vi "前面板对象常用属性.vi"() -> ()   [LabVIEW 2010]
panel:
  out "1号罐图标大小":cluster{"宽":u32, "高":u32}
  in  "停止":bool
  in  "键盘焦点":bool
  in  "极限设定":dbl(slide)=5.252525252525253 scale=0.0..10.0
  out "4号罐液位":dbl(slide)=6.506024096385542 scale=0.0..10.0
  in  "可用":i32(listbox)
  in  "3号罐液位":dbl(slide)=6.506024096385542 scale=0.0..10.0
  in  "不闪烁   闪烁":bool=TRUE
  in  "2号罐液位":dbl(slide)=6.385542168674699 scale=0.0..10.0
  in  "1号罐液位":dbl(slide)=6.265060240963855 scale=0.0..10.0
  in  "不可见   可见":bool=TRUE
  # "取消    设定"
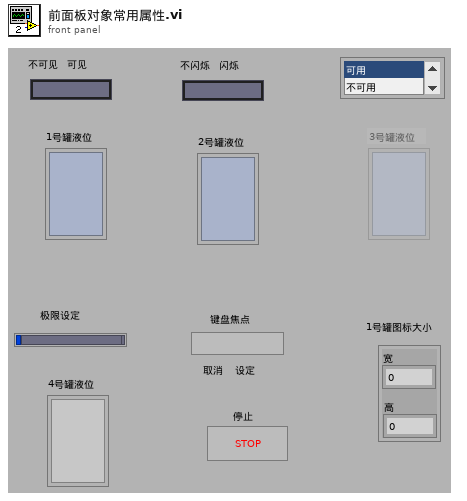
[diagram p1: front panel]
types:
  T1 = typedef "LVBoundsTypeDef.ctl" = cluster{"Width":u32, "Height":u32}
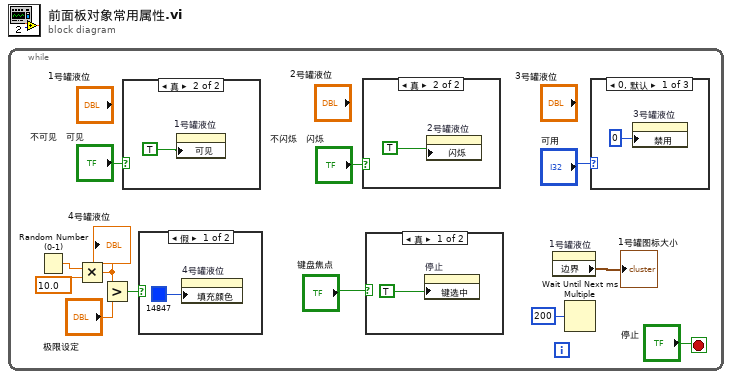
[diagram p0: block diagram]
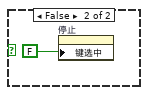
[diagram p2: hidden frame]
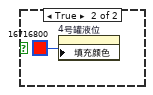
[diagram p3: hidden frame]
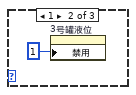
[diagram p4: hidden frame]
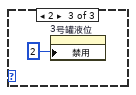
[diagram p5: hidden frame]
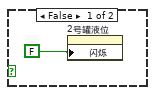
[diagram p6: hidden frame]
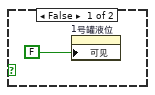
[diagram p7: hidden frame]
diagram:
  n1 = while {
    stop <- "停止" stop-if-true
    n2 = Random Number (0-1)() -> (number: 0 to 1=w7:dbl)
    n3 = Multiply(x=w7, y=10.0) -> (x*y=w5:dbl)
    "4号罐液位" <- w5
    n4 = Greater?(x=w5, y="极限设定") -> (0:w8:bool)
    n5 = case shown="真" "不可见   可见" {
      frame False {
        n6 = property on="1号罐液位" class="Slide (严格)"("可见"=FALSE) -> ()  [unwired: 2 in, 2 out]
      }
      frame True {
        n7 = property on="1号罐液位" class="Slide (严格)"("可见"=TRUE) -> ()  [unwired: 2 in, 2 out]
      }
    }
    n8 = case shown="假" w8 {
      frame False {
        n9 = property on="4号罐液位" class="Slide (严格)"("填充颜色"=u32 14847) -> ()  [unwired: 2 in, 2 out]
      }
      frame True {
        n10 = property on="4号罐液位" class="Slide (严格)"("填充颜色"=u32 16716800) -> ()  [unwired: 2 in, 2 out]
      }
    }
    n11 = case shown="真" "不闪烁   闪烁" {
      frame False {
        n12 = property on="2号罐液位" class="Slide (严格)"("闪烁"=FALSE) -> ()  [unwired: 2 in, 2 out]
      }
      frame True {
        n13 = property on="2号罐液位" class="Slide (严格)"("闪烁"=TRUE) -> ()  [unwired: 2 in, 2 out]
      }
    }
    n14 = case shown="真" "键盘焦点" {
      frame True {
        n15 = property on="停止" class="Bool"("键选中"=TRUE) -> ()  [unwired: 2 in, 2 out]
      }
      frame False {
        n16 = property on="停止" class="Bool"("键选中"=FALSE) -> ()  [unwired: 2 in, 2 out]
      }
    }
    n17 = property on="1号罐液位" class="Slide (严格)"() -> ("边界"=→"1号罐图标大小":T1)  [unwired: 2 in, 2 out]
    n18 = Wait Until Next ms Multiple(millisecond multiple=u32 200) -> ()  [unwired: 1 out]
    n19 = case shown="0, 默认" "可用" {
      frame 0, Default {
        n20 = property on="3号罐液位" class="Slide (严格)"("禁用"=0) -> ()  [unwired: 2 in, 2 out]
      }
      frame 1 {
        n21 = property on="3号罐液位" class="Slide (严格)"("禁用"=1) -> ()  [unwired: 2 in, 2 out]
      }
      frame 2 {
        n22 = property on="3号罐液位" class="Slide (严格)"("禁用"=2) -> ()  [unwired: 2 in, 2 out]
      }
    }
  }
